vi "Do.vi"(8 "error in (no error)":errorcluster, 10 "Actor in":refnum<class "Actor.lvclass">, 11 "fire actor ui Msg":refnum<class "fire actor ui Msg.lvclass">) -> (0 "error out":errorcluster, 2 "Actor out":refnum<class "Actor.lvclass">)   [LabVIEW 2020, in "Template.lvlib" / "fire actor ui Msg.lvclass"]
doc: "This VI delivers the message to the actor by calling the appropriate method(s) on the actor."
uses:
  fire actor ui Msg.lvclass
  <vilib>/ActorFramework/Actor/Actor.lvclass
  template/Template.lvclass
  C:/Program Files/National Instruments/LabVIEW 2020/vi.lib/ActorFramework/Actor/Actor.lvclass
  9ef47adc-f318-494c-9b8b-6df3216d6863.vi
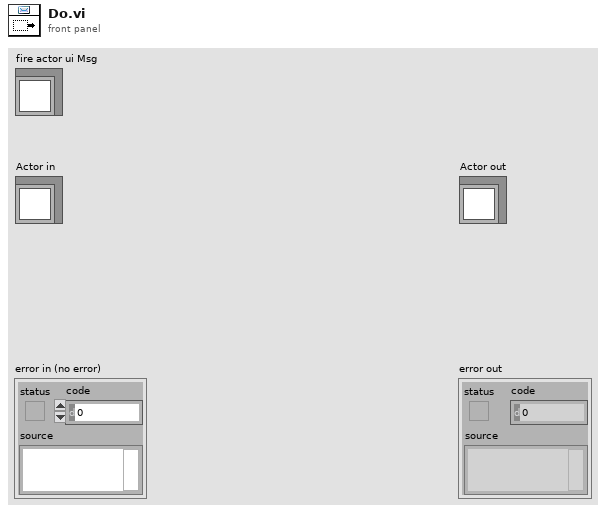
[diagram p1: front panel]
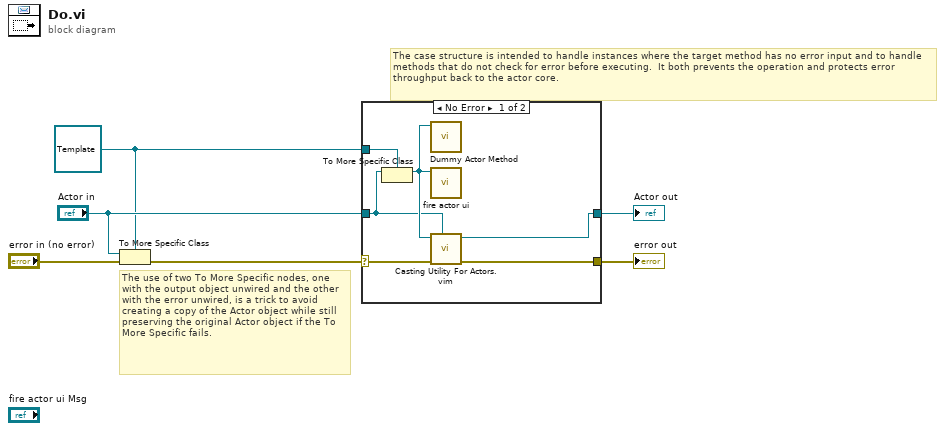
[diagram p0: block diagram]
diagram:
  w1 = refnum<class "Template.lvclass"> refnum ("Actor in")
  # "The use of two To More Specific nodes, one with the output object unwired and the other with the error unwired, is a trick to avoid creating a copy of the Actor object while still preserving the original Actor object if the To More Specific fails."
  # "The case structure is intended to handle instances where the target method has no error input and to handle methods that do not check for error before executing.  It both prevents the operation and protects error throughput back to the actor core."
  n1 = To More Specific Class(target class=w1, reference="Actor in", error in="error in (no error)") -> (error out=w5:errorcluster)  [unwired: 1 out]
  n2 = case shown="No Error" w5 {
    selector: w5 -> [w12 w14]
    tunnel: [w7 w14] -> w4
    tunnel: [w8 w13] -> w3
    tunnel: "Actor in" -> [w9 w13]
    tunnel: w1 -> [w10 _]
    frame No Error {
      n3 = To More Specific Class(target class=w10, reference=w9) -> (specific class reference=w11:refnum<class "Template.lvclass">)  [unwired: 1 in, 1 out]
      n4 = call <resource>:"Dummy Actor Method.vi"("Actor in"=w11) -> ()  [unwired: 9 in, 2 out]
      n5 = call "fire actor ui.vi"("Template in"=w11) -> ()  [unwired: 11 in]
      n6 = call "Casting Utility For Actors.vim"("type"=w9, "error in (no error)"=w12, "Actor in"=w11) -> ("error out"=w7:errorcluster, "Actor out"=w8:refnum<class "Actor.lvclass">)  [unwired: 7 in]
    }
    frame Error {
      # "If type check fails, pass the original object out again."
    }
  }
  "error out" <- w4
  "Actor out" <- w3
